vi "Analyze Vacuum Transition.vi"(7 "Vacuum Specs":T1, 9 "Data After":T2[](array[typedef]), 10 "Cart Array":bool[](array[boolean]), 11 "Data Before":T2[](array[typedef])) -> (1 "TransitionPass":bool[](array[boolean]), 2 "VacLevelPass":bool[](array[boolean]), 3 "Analysis":T3[](array[typedef]))   [LabVIEW 2018]
uses:
  Vacuum Test.ctl
  Vacuum Output.ctl
  Vacuum Specs.ctl
panel:
  out "StabilityPass":bool[](array[boolean])
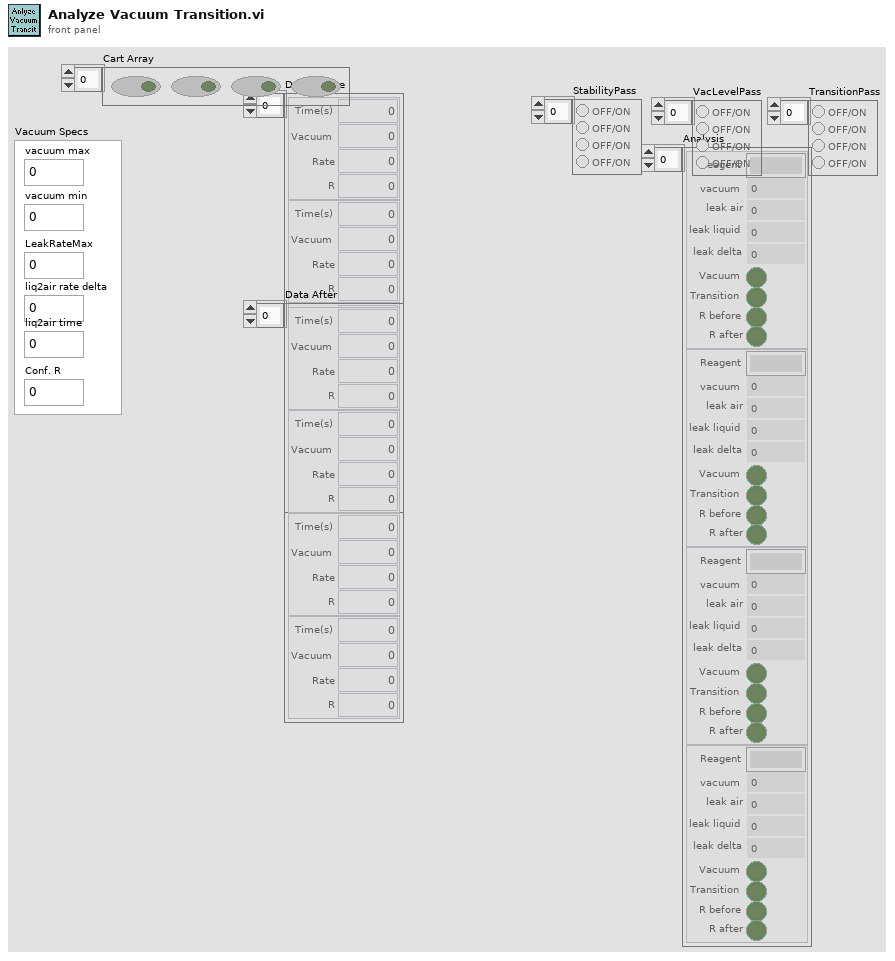
[diagram p1: front panel]
types:
  T1 = typedef "Vacuum Specs.ctl" = cluster{"vacuum max":dbl, "vacuum min":dbl, "liq2air rate delta":dbl, "liq2air time":dbl, "Conf. R":dbl, "LeakRateMax":dbl}
  T2 = typedef "Vacuum Output.ctl" = cluster{"Time(s)":dbl, "Vacuum":dbl, "Rate":dbl, "R":dbl}
  T3 = typedef "Vacuum Test.ctl" = cluster{"vacuum":dbl, "leak air":dbl, "leak liquid":dbl, "leak delta":dbl, "Transition":bool, "Vacuum":bool, "R before":bool, "R after":bool, "Reagent":string}
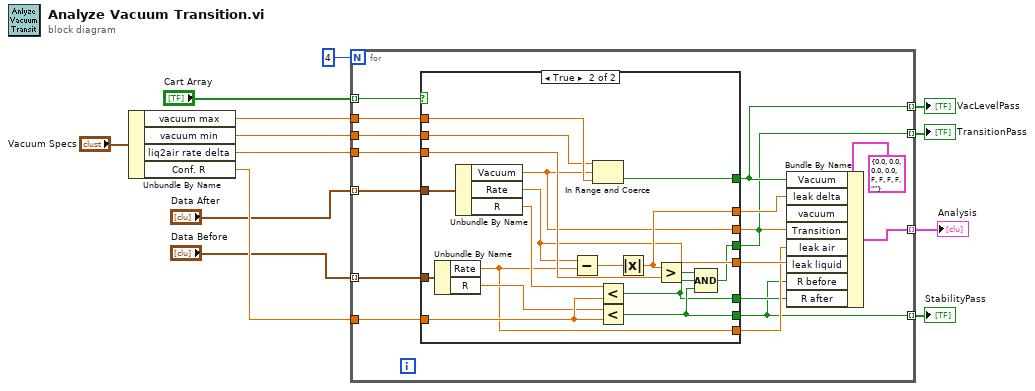
[diagram p0: block diagram]
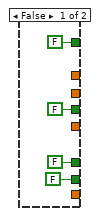
[diagram p2: hidden frame]
diagram:
  n1 = Unbundle By Name("Vacuum Specs") -> ("vacuum max"=w7:dbl, "vacuum min"=w8:dbl, "liq2air rate delta"=w11:dbl, "Conf. R"=w13:dbl)
  n2 = for {
    N: 4 -> [_]
    tunnel: "Data After" -> [w25] mode=indexing
    tunnel: w7 -> [w30]
    tunnel: w8 -> [w29]
    tunnel: "Data Before" -> [w24] mode=indexing
    tunnel: w11 -> [w27]
    tunnel: [w26] -> w12 mode=indexing
    tunnel: w13 -> [w21]
    tunnel: [w20] -> w3 mode=indexing
    tunnel: [w18] -> w2 mode=indexing
    tunnel: "Cart Array" -> [w19] mode=indexing
    tunnel: [w14] -> w1 mode=indexing
    n3 = case shown="True" w19 {
      tunnel: w30 -> [_ w52]
      tunnel: w29 -> [_ w51]
      tunnel: w27 -> [_ w50]
      tunnel: w25 -> [_ w49]
      tunnel: w24 -> [_ w48]
      tunnel: [_ w47] -> w23
      tunnel: [_ w46] -> w22
      tunnel: [_ w45] -> w17
      tunnel: w21 -> [_ w44]
      tunnel: [FALSE w39] -> w20
      tunnel: [FALSE w38] -> w18
      tunnel: [FALSE w37] -> w14
      tunnel: [_ w36] -> w16
      tunnel: [FALSE w35] -> w15
      frame False {
      }
      frame True {
        n4 = Unbundle By Name(w48) -> ("Rate"=w36:dbl, "R"=w41:dbl)
        n5 = Unbundle By Name(w49) -> ("Vacuum"=w46:dbl, "Rate"=w45:dbl, "R"=w42:dbl)
        n6 = Subtract(x=w45, y=w36) -> (x-y=w43:dbl)
        n7 = In Range and Coerce(upper limit=w51, x=w46, lower limit=w52) -> (In Range?=w39:bool)  [unwired: 1 out]
        n8 = Less?(x=w42, y=w44) -> (x < y?=w35:bool)
        n9 = Less?(x=w41, y=w44) -> (x < y?=w37:bool)
        n10 = Absolute Value(x=w43) -> (abs(x)=w47:dbl)
        n11 = Greater?(x=w47, y=w50) -> (0:w40:bool)
        n12 = Compound Arithmetic op=AND(w40, w35, w37) -> (w38:bool)
      }
    }
    n13 = Bundle By Name(cluster=T3 {"vacuum"=0.0, "leak air"=0.0, "leak liquid"=0.0, "leak delta"=0.0, "Transition"=FALSE, "Vacuum"=FALSE, "R before"=FALSE, "R after"=FALSE, "Reagent"=""} ("Result"), "Vacuum"=w20, "leak delta"=w23, "vacuum"=w22, "Transition"=w18, "leak air"=w16, "leak liquid"=w17, "R before"=w14, "R after"=w15) -> (w26:T3)
  }
  "Analysis" <- w12
  "VacLevelPass" <- w3
  "TransitionPass" <- w2
  "StabilityPass" <- w1
